vi "LED Indicater Logic.vi"() -> (4 "Read4Gear":bool, 6 "Traction":bool, 8 "Intake":bool, 10 "Brakes":bool, 15 "Hood Up":bool)   [LabVIEW 2016]
uses:
  Robot Code/Robot Global Data.vi
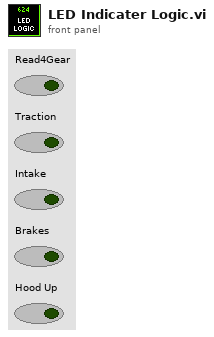
[diagram p1: front panel]
types:
  T1 = typedef "Shooter Control Cluster'.ctl" = cluster{"Shooter Modes":T2, "Shooter Commands":T3, "manUEL Control Cluster":T4, "Shot Type":T5}
  T2 = typedef "Shooter Modes.ctl" = enum16{"Auto", "Manual"}
  T3 = typedef "Shooter Commands.ctl" = enum16{"Idle ", "Warmup ", "Shoot"}
  T4 = typedef "Manual Shoot Cluster.ctl" = cluster{"Shot RPM":dbl, "Wait Time":dbl, "da HOOD?":bool}
  T5 = typedef "Shot Type.ctl" = enum16{"Vision Shot", "Dist Shot", "Key Shot"}
  T6 = typedef "Intake Control Cluster.ctl" = cluster{"Intake Modes":T7, "Auto Ball Commands":T8, "Intake Current Trip States":T9, "Proposed Intake Power":dbl, "Fill Hopper?":bool, "Get Gear?":bool, "Auto Gear Commands":T10, "Proposed Outake Power":dbl, "Power Constant":dbl, "Resistance Tolerance":dbl, "Power Tolerance":dbl, "Current Correct":dbl}
  T7 = typedef "Intake Modes.ctl" = enum16{"Manual", "Auto"}
  T8 = typedef "Intake Auto States.ctl" = enum16{"Outtake Ball", "Current Tripped ", "Idle", "Load Ball"}
  T9 = typedef "Intake Trip States.ctl" = enum16{"Normal", "Backward Tripped", "Forward Tripped"}
  T10 = typedef "Auto Gear State.ctl" = enum16{"Idle ", "Intake "}
  T11 = typedef "Drivetrain Status Cluster.ctl" = cluster{"Drivetrain Mode":enum16{"Manual", "Gyro Steer"}, "Y (Throttle)":dbl, "X (Steer)":dbl, "Z (Strafe)":dbl, "Heading Target":dbl, "Center Piston Down?":bool, "Traction?":bool, "Gyro Steer Finished?":bool, "Distance Drive Finished?":bool, "Gyro":dbl, "Distance Target":dbl, "Y Max Output":dbl, "Y Min Output":dbl, "X Max Output":dbl, "X Min Output":dbl, "Z Max Output":dbl, "Z Min Output":dbl, "Translation Target":dbl, "Translation Drive Finished?":bool}
  T12 = typedef "Intake Status Cluster.ctl" = cluster{"Roller Speed":dbl, "Intake Modes":T7, "Intake Auto Commands":T8, "Backward Tripped?":bool, "Forward Tripped?":bool, "Filling Hopper?":bool, "Intake Current Trip States":T9, "Getting Gear?":bool}
  T13 = typedef "Drivetrain Command Cluster.ctl" = cluster{"Drivetrain Mode":T14, "Heading Target":dbl, "Turn Power":dbl, "Y Power":dbl, "Center Piston Down?":bool, "Traction?":bool, "Strafe Power":dbl, "Zero Gyro":bool, "Distance Target":dbl, "Strafe Correct":bool, "Y Max Output":dbl, "Y Min Output":dbl, "X Max Output":dbl, "X Min Output":dbl, "Z Max Output":dbl, "Z Min Output":dbl, "Z Target":dbl, "Brake?":bool}
  T14 = typedef "Drivetrain Mode.ctl" = enum16{"Manual", "Gyro Steer", "Distance Drive", "Translate Drive", "PID Drive"}
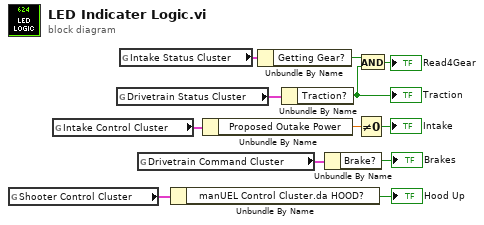
[diagram p0: block diagram]
diagram:
  n1 = global read "Robot Global Data.vi" "Shooter Control Cluster"() -> (w11:T1)
  n2 = global read "Robot Global Data.vi" "Intake Control Cluster"() -> (w9:T6)
  n3 = global read "Robot Global Data.vi" "Drivetrain Status Cluster"() -> (w12:T11)
  n4 = global read "Robot Global Data.vi" "Intake Status Cluster"() -> (w4:T12)
  n5 = global read "Robot Global Data.vi" "Drivetrain Command Cluster"() -> (w6:T13)
  n6 = Unbundle By Name(w11) -> ("manUEL Control Cluster.da HOOD?"=→"Hood Up":bool)
  n7 = Unbundle By Name(w9) -> ("Proposed Outake Power"=w8:dbl)
  n8 = Unbundle By Name(w4) -> ("Getting Gear?"=w2:bool)
  n9 = Unbundle By Name(w12) -> ("Traction?"=w1:bool)
  "Traction" <- w1
  n10 = Unbundle By Name(w6) -> ("Brake?"=→"Brakes":bool)
  n11 = Not Equal To 0?(x=w8) -> (x != 0?=→"Intake":bool)
  n12 = And(x=w2, y=w1) -> (x .and. y?=→"Read4Gear":bool)
